vi "dbServerConnect.vi"   [LabVIEW 2025]
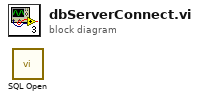
[diagram p0: block diagram]
diagram:
  n1 = call <vilib>:"SQL Open.vi"() -> ()  [unwired: 18 in, 2 out]
